vi "RecursiveDependenceies.vi"(8 "error in (no error)":errorcluster, 10 "Object":variant, 11 "JSON Schema in":string) -> (0 "error out":errorcluster, 3 "JSON Schema out":string)   [LabVIEW 2019, in "JSON-Schema.lvlib"]
uses:
  JSON-Schema.lvlib
  <vilib>/JDP Science/JSONtext/Next JSON Value.vi
  <vilib>/JDP Science/JSONtext/String Subset.vi
  <vilib>/JDP Science/JSONtext/Parsing/Advance past next JSON Value (inlined COPY).vi
  <vilib>/JDP Science/JSONtext/Parsing/Advance past whitespace.vi
  <vilib>/JDP Science/JSONtext/Parsing/Advance past String.vi
  <vilib>/JDP Science/JSONtext/Parsing/Advance past Number.vi
  <vilib>/JDP Science/JSONtext/Parsing/Advance past Line Ending.vi
  <vilib>/JDP Science/JSONtext/Parsing/Parse Full Path or Item Name.vi
  <vilib>/JDP Science/JSONtext/Parsing/Advance past Array.vi
  <vilib>/JDP Science/JSONtext/Parsing/Advance past Object.vi
  <vilib>/JDP Science/JSONtext/support/Error Cluster From Code.vi
  <vilib>/JDP Science/JSONtext/Offset/Find Item Locations by Path.vi
  <vilib>/JDP Science/JSONtext/JSONtext.lvlib
  <vilib>/Utility/Data Type/NI_Data Type.lvlib
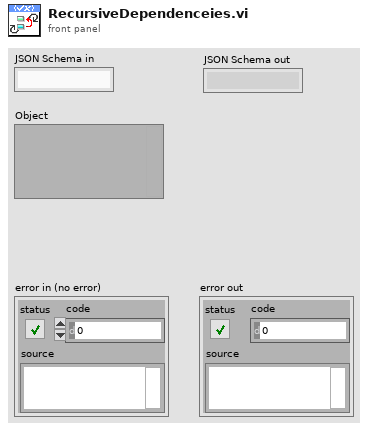
[diagram p1: front panel]
types:
  T1 = typedef "NI_Data Type.lvlib/Data Type.ctl" = enum8{"Invalid Type", "Void", "I8", "I16", "I32", "I64", "U8", "U16", "U32", "U64", "Single Float", "Double Float", "Extended Float", "Single Complex", "Double Complex", "Extended Complex", "Enum U8", "Enum U16", "Enum U32", "Enum U64", "Single Float With Unit", "Double Float With Unit", "Extended Float With Unit", "Single Complex with Unit", "Double Complex with Unit", "Extended Complex with Unit", "Boolean", "String", "Path", "Picture", "Tag", "Array", "Cluster", "Variant", "LV Variant", "Waveform", "Timestamp", "Digital Waveform", "Digital Data", "ExpressData", "Refnum", "External Data", "VI", "Poly VI", "LabVIEW Class Instance", "Fixed Point", "Set Collection", "Map Collection"}
  T2 = typedef "NI_Data Type.lvlib/Type Definition Info.ctl" = cluster{"Name":string, "Timestamp":u32}
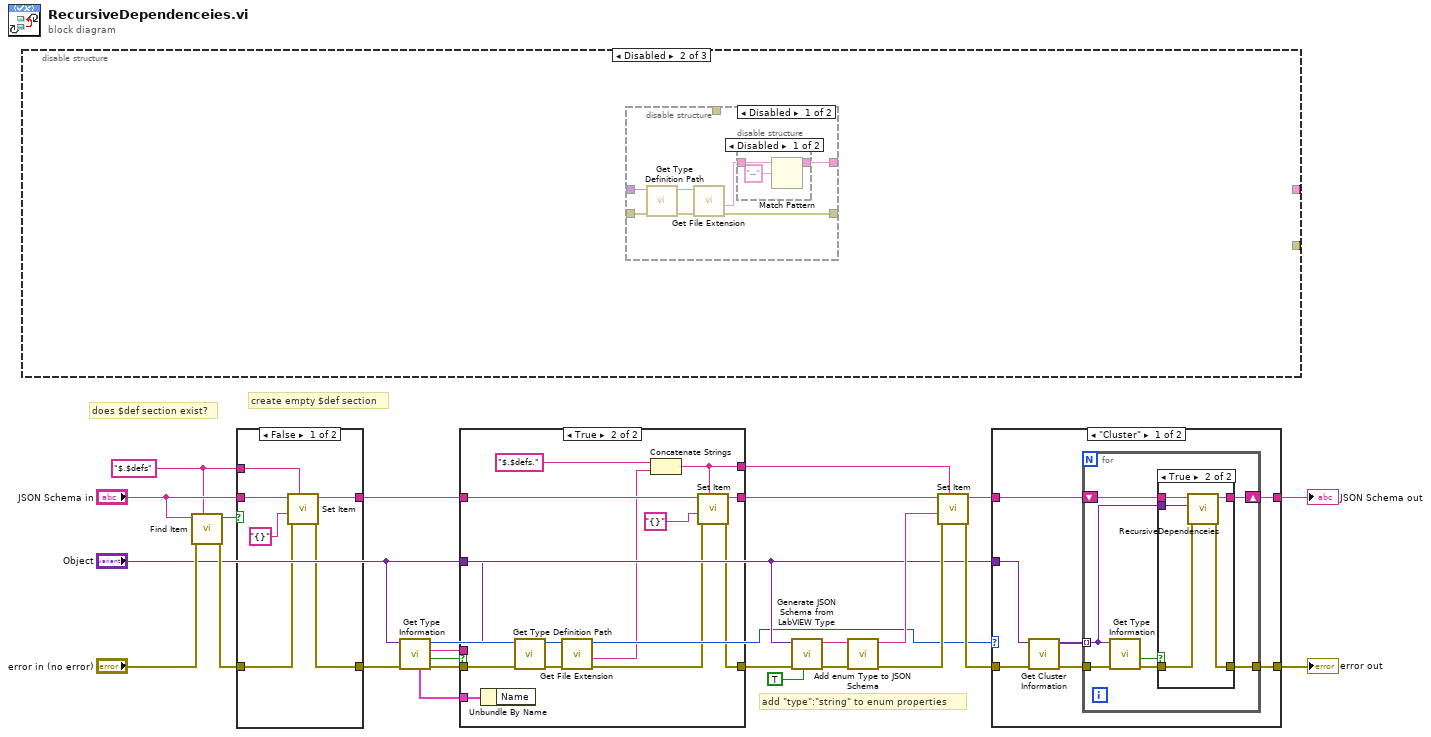
[diagram p0: block diagram]
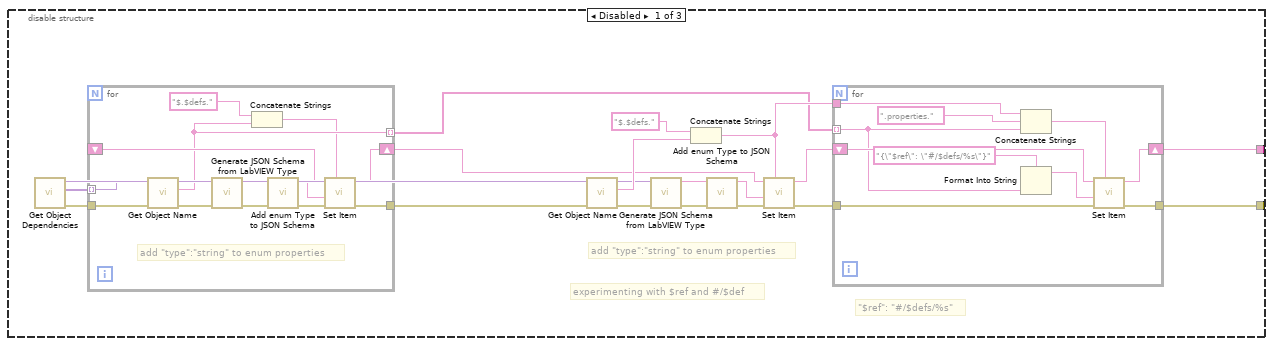
[diagram p6: hidden frame]
diagram:
  w20 = "$.$defs" ("$Path or Item Name")
  # "add \"type\":\"string\" to enum properties"
  # "create empty $def section"
  # "does $def section exist?"
  n1 = disable-structure shown="Disabled" {
    disable-tunnel: [w27 _ _] -> _
    disable-tunnel: [w26 _ _] -> _
    frame Disabled {
      # "experimenting with $ref and #/$def"
      # "\"$ref\": \"#/$defs/%s\""
      # "add \"type\":\"string\" to enum properties"
      n2 = call "Get Object Dependencies.vi"() -> ("error out"=w43:errorcluster, "values"=w44:variant[], "Variant"=w30:variant)  [unwired: 9 in]
      n3 = for {
        tunnel: [w65] -> w29
        shift-right: [w66] -> w28
        shift-left: [w62] -> w45
        tunnel: w44 -> [w60] mode=indexing
        tunnel: w43 -> [w59]
        tunnel: [w57] -> w31 mode=indexing
        # "add \"type\":\"string\" to enum properties"
        n4 = call "Get Object Name.vi"("error in (no error)"=w59, "Object"=w60) -> ("error out"=w61:errorcluster, "name"=w57:string, "Variant"=w63:variant)  [unwired: 7 in]
        n5 = call <vilib>:"Generate JSON Schema from LabVIEW Type.vi"("error in (no error)"=w61, "Variant"=w63) -> ("error out"=w69:errorcluster, "JSON Schema"=w68:string)  [unwired: 8 in]
        n6 = Concatenate Strings("$.$defs." ("format string"), w57) -> (w56:string)
        n7 = call "Add enum Type to JSON Schema.vi"("error in (no error)"=w69, "JSON Schema in"=w68) -> ("error out"=w67:errorcluster, "JSON Schema out"=w64:string)  [unwired: 8 in]
        n8 = call <vilib>:"Set Item.vi"("$Path or Item Name"=w56, "error in (no error)"=w67, "JSON to Insert"=w64, "JSON"=w62) -> ("error out"=w65:errorcluster, "<JSON>"=w66:string)  [unwired: 4 in, 1 out]
      }
      n9 = call "Get Object Name.vi"("error in (no error)"=w29, "Object"=w30) -> ("error out"=w38:errorcluster, "name"=w39:string, "Variant"=w37:variant)  [unwired: 7 in]
      n10 = call <vilib>:"Generate JSON Schema from LabVIEW Type.vi"("error in (no error)"=w38, "Variant"=w37) -> ("error out"=w33:errorcluster, "JSON Schema"=w34:string)  [unwired: 8 in]
      n11 = Concatenate Strings("$.$defs." ("format string"), w39) -> (w41:string)
      n12 = call "Add enum Type to JSON Schema.vi"("error in (no error)"=w33, "JSON Schema in"=w34) -> ("error out"=w35:errorcluster, "JSON Schema out"=w36:string)  [unwired: 8 in]
      n13 = call <vilib>:"Set Item.vi"("$Path or Item Name"=w41, "error in (no error)"=w35, "JSON to Insert"=w36, "JSON"=w28) -> ("error out"=w40:errorcluster, "<JSON>"=w42:string)  [unwired: 4 in, 1 out]
      n14 = for {
        tunnel: [w54] -> w27
        shift-right: [w55] -> w26
        shift-left: w42 -> [w53]
        tunnel: w31 -> [w48] mode=indexing
        tunnel: w40 -> [w51]
        tunnel: w41 -> [w46]
        n15 = Concatenate Strings(w46, ".properties." ("string"), w48) -> (w52:string)
        n16 = Format Into String(format string="{\"$ref\": \"#/$defs/%s\"}", w48) -> (resulting string=w49:string)  [unwired: 2 in, 1 out]
        n17 = call <vilib>:"Set Item.vi"("$Path or Item Name"=w52, "error in (no error)"=w51, "JSON to Insert"=w49, "JSON"=w53) -> ("error out"=w54:errorcluster, "<JSON>"=w55:string)  [unwired: 4 in, 1 out]
      }
    }
    frame Disabled {
      n18 = disable-structure shown="Disabled" {
        disable-tunnel: _ -> [w76 _]
        disable-tunnel: [w75 _] -> _
        disable-tunnel: _ -> [w72 w81]
        disable-tunnel: [w70 _] -> _
        disable-tunnel: [_ w81] -> _
        frame Disabled {
          n19 = call <vilib>:"Get Type Definition Path.vi"("error in (no error)"=w72, "variant"=w76) -> ("error out"=w73:errorcluster, "type definition path"=w74:path)  [unwired: 8 in]
          n20 = call <vilib>:"Get File Extension.vi"("error in (no error)"=w73, "file"=w74) -> ("error out"=w70:errorcluster, "filename without extension"=w71:string)  [unwired: 5 in, 3 out]
          n21 = disable-structure shown="Disabled" {
            disable-tunnel: [w78 w80] -> w75
            disable-tunnel: w71 -> [w77 w80]
            frame Disabled {
              n22 = Match Pattern(string=w77, regular expression="--") -> (before substring=w78:string)  [unwired: 1 in, 3 out]
            }
            frame Enabled {
            }
          }
        }
        frame Enabled {
        }
      }
    }
    frame Enabled {
    }
  }
  n23 = call <vilib>:"Find Item.vi"("$Path or Item Name"=w20, "error in (no error)"="error in (no error)", "JSON"="JSON Schema in") -> ("error out"=w18:errorcluster, "Found"=w17:bool)  [unwired: 5 in, 2 out]
  n24 = case shown="False" w17 {
    tunnel: [w86 w88] -> w25
    tunnel: [w85 w89] -> w15
    tunnel: "JSON Schema in" -> [w84 w89]
    tunnel: w20 -> [w83 _]
    tunnel: w18 -> [w82 w88]
    frame False {
      n25 = call <vilib>:"Set Item.vi"("$Path or Item Name"=w83, "error in (no error)"=w82, "JSON to Insert"="{}", "JSON"=w84) -> ("error out"=w86:errorcluster, "<JSON>"=w85:string)  [unwired: 4 in, 1 out]
    }
    frame True {
    }
  }
  n26 = call <vilib>:"Get Type Information.vi"("error in (no error)"=w25, "variant"="Object") -> ("error out"=w23:errorcluster, "type definition"=w22:bool, "name"=w24:string, "type"=w2:T1, "type definition info"=w16:T2)  [unwired: 5 in]
  n27 = case shown="True" w22 {
    tunnel: w23 -> [w92 w94]
    tunnel: w24 -> [w90 _]
    tunnel: [w92 w100] -> w7
    tunnel: w16 -> [_ w105]
    tunnel: w15 -> [w91 w102]
    tunnel: [w91 w101] -> w4
    tunnel: [w90 w99] -> w5
    tunnel: "Object" -> [_ w96]
    frame False {
    }
    frame True {
      n28 = Unbundle By Name(w105) -> ()  [unwired: 1 out]
      n29 = call <vilib>:"Get Type Definition Path.vi"("error in (no error)"=w94, "variant"=w96) -> ("error out"=w97:errorcluster, "type definition path"=w98:path)  [unwired: 8 in]
      n30 = call <vilib>:"Get File Extension.vi"("error in (no error)"=w97, "file"=w98) -> ("error out"=w95:errorcluster, "filename without extension"=w93:string)  [unwired: 5 in, 3 out]
      n31 = Concatenate Strings("$.$defs." ("$Path or Item Name"), w93) -> (w99:string)
      n32 = call <vilib>:"Set Item.vi"("$Path or Item Name"=w99, "error in (no error)"=w95, "JSON to Insert"="{}", "JSON"=w102) -> ("error out"=w100:errorcluster, "<JSON>"=w101:string)  [unwired: 4 in, 1 out]
    }
  }
  n33 = call <vilib>:"Generate JSON Schema from LabVIEW Type.vi"("Strict Clusters"=TRUE, "error in (no error)"=w7, "Variant"="Object") -> ("error out"=w11:errorcluster, "JSON Schema"=w12:string)  [unwired: 7 in]
  n34 = call "Add enum Type to JSON Schema.vi"("error in (no error)"=w11, "JSON Schema in"=w12) -> ("error out"=w9:errorcluster, "JSON Schema out"=w10:string)  [unwired: 8 in]
  n35 = call <vilib>:"Set Item.vi"("$Path or Item Name"=w5, "error in (no error)"=w9, "JSON to Insert"=w10, "JSON"=w4) -> ("error out"=w6:errorcluster, "<JSON>"=w1:string)  [unwired: 4 in, 1 out]
  n36 = case shown="\"Cluster\"" w2 {
    tunnel: "Object" -> [w111 _]
    tunnel: w6 -> [w112 w128]
    tunnel: [w107 w128] -> w14
    tunnel: w1 -> [w110 w127]
    tunnel: [w106 w127] -> w13
    frame "Cluster" {
      n37 = call <vilib>:"Get Cluster Information.vi"("error in (no error)"=w112, "variant"=w111) -> ("error out"=w108:errorcluster, "cluster elements"=w109:variant[])  [unwired: 8 in]
      n38 = for {
        tunnel: w109 -> [w114] mode=indexing
        shift-right: [w118] -> w106
        shift-left: w110 -> [w119]
        tunnel: w108 -> [w115]
        tunnel: [w117] -> w107
        n39 = call <vilib>:"Get Type Information.vi"("error in (no error)"=w115, "variant"=w114) -> ("error out"=w116:errorcluster, "type definition"=w113:bool)  [unwired: 5 in, 3 out]
        n40 = case shown="True" w113 {
          tunnel: w119 -> [w120 w126]
          tunnel: [w120 w125] -> w118
          tunnel: [w121 w124] -> w117
          tunnel: w116 -> [w121 w123]
          tunnel: w114 -> [_ w122]
          frame False {
          }
          frame True {
            n41 = call "RecursiveDependenceies.vi"("error in (no error)"=w123, "Object"=w122, "JSON Schema in"=w126) -> ("error out"=w124:errorcluster, "JSON Schema out"=w125:string)  [unwired: 7 in]
          }
        }
      }
    }
    frame Default {
    }
  }
  "error out" <- w14
  "JSON Schema out" <- w13
